vi "qOAC.vi"(0 "System no.":i32=1 min=1 max=4 step=1, 2 "Axes to query":string[](array[string]), 3 "All axes?":bool, 4 "Axis identifier?":bool=TRUE, 5 "error in":errorcluster) -> (14 "Acceleration":dbl[](array[numeric]) format="%.6f", 19 "error out":errorcluster)   [LabVIEW 2020]
doc: "Returns open-loop acceleration setting for specified axes.\n\nE-861, E-874: If All axes? = TRUE, then Axis identifier? can be FALSE. Velocity unit is steps/s²."
panel:
  # "Returns open-loop acceleration setting for specified axes."
  # "If all axes: use"
  # "Query"
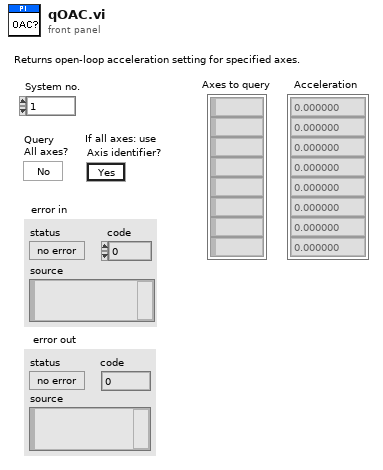
[diagram p1: front panel]
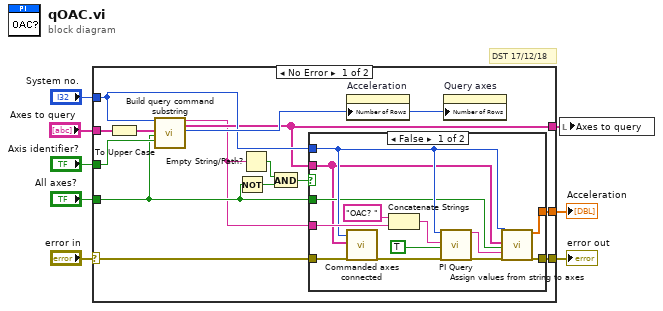
[diagram p0: block diagram]
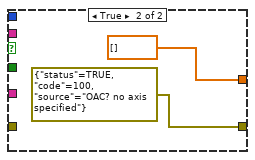
[diagram p2: hidden frame]
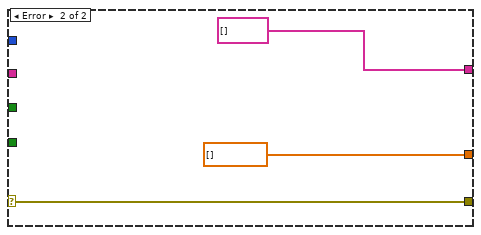
[diagram p3: hidden frame]
diagram:
  # "DST 17/12/18"
  n1 = case shown="No Error" "error in" {
    selector: "error in" -> [w13 w39]
    tunnel: [w22 dbl[] [] ("Values")] -> w8
    tunnel: "Axes to query" -> [w21 _]
    tunnel: [w20 w39] -> w6
    tunnel: "Axis identifier?" -> [w18 _]
    tunnel: "System no." -> [w16 _]
    tunnel: "All axes?" -> [w15 _]
    tunnel: [w12 string[] [] ("Axes to query out")] -> w1
    frame No Error {
      n2 = To Upper Case(1:w21) -> (0:w19:string[])
      n3 = call "Build query command substring.vi"("System no."=w16, "Axes to query in"=w19, "Query\nAll axes?"=w15, "For all axes: use\nAxis identifier?"=w18) -> ("Command substring"=w10:string, "Axes to query out"=w12:string[], "Number of rows"=w17:u32)  [unwired: 2 in, 11 out]
      n4 = Not(x=w15) -> (.not. x?=w14:bool)
      n5 = Empty String/Path?(string/path=w10) -> (empty?=w9:bool)
      n6 = And(x=w9, y=w14) -> (x .and. y?=w11:bool)
      n7 = case shown="False" w11 {
        tunnel: [w32 dbl[] [] ("Values")] -> w22
        tunnel: [w23 errorcluster {"status"=TRUE, "code"=100, "source"="OAC? no axis specified"} ("error out")] -> w20
        tunnel: w10 -> [w31 _]
        tunnel: w16 -> [w30 _]
        tunnel: w15 -> [w29 _]
        tunnel: w13 -> [w27 _]
        tunnel: w12 -> [w26 _]
        frame False {
          n8 = call "Commanded axes connected.vi"("System no."=w30, "Commanded axes"=w26, "error in"=w27) -> ("error out"=w28:errorcluster)  [unwired: 1 in, 15 out]
          n9 = Concatenate Strings("OAC? ", w31) -> (w33:string)
          n10 = call "PI Query.vi"("System no."=w30, "String to send"=w33, "Attach termination char.?"=TRUE ("Attach Linefeed?"), "error in"=w28) -> ("String read"=w24:string, "error out"=w25:errorcluster)  [unwired: 3 in, 11 out]
          n11 = call "Assign values from string to axes.vi"("System no."=w30, "Queried axes"=w26, "All axes queried?"=w29, "Input String"=w24, "error in"=w25) -> ("Values"=w32:dbl[], "error out"=w23:errorcluster)  [unwired: 4 in, 9 out]
        }
        frame True {
        }
      }
      n12 = property on="Acceleration" class="Arr (strict)"("Number of Rows"=w17) -> ()  [unwired: 2 in, 2 out]
      n13 = property on="Query axes" class="Arr (strict)"("Number of Rows"=w17) -> ()  [unwired: 2 in, 2 out]
    }
    frame Error {
    }
  }
  "error out" <- w6
  "Acceleration" <- w8
  n14 = local write "Axes to query"(w1) -> ()
